vi "onCreated.vi"(8 "error in (no error)":errorcluster, 11 "Generator":refnum<class "Generator.lvclass">) -> (0 "error out":errorcluster, 3 "Generator out":refnum<class "Generator.lvclass">)   [LabVIEW 2019, in "Generator.lvclass"]
uses:
  Generator.lvclass
  <vilib>/JKI/JKI SMO/SMO/SMO.lvclass
panel:
  # "For instructions on how to use the JKI State Machine Objects, examples and video tutorials, visit:\nhttp://jki.net/state-machine-objects/\n\nJKI State Machine Objects™\nhttp://jki.net/state-machine-objects/\nCopyright (C) 2005-2015, JKI <info@jki.net>\nALL RIGHTS RESERVED"
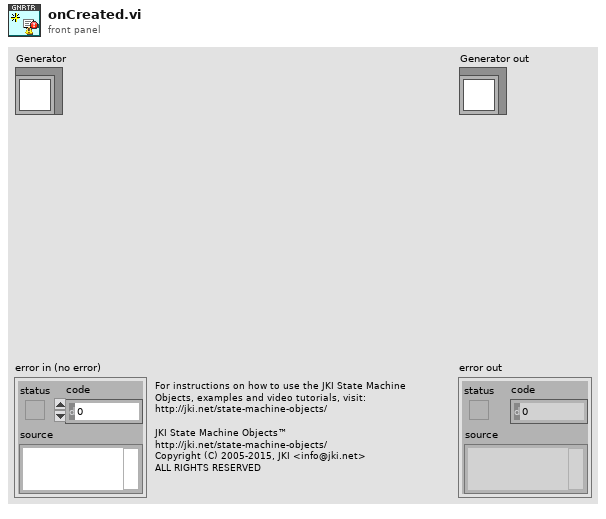
[diagram p1: front panel]
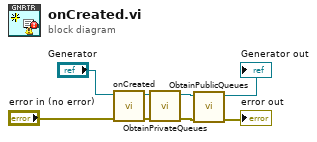
[diagram p0: block diagram]
diagram:
  n1 = call-parent "onCreated.vi"("error in (no error)"="error in (no error)", "SMO"="Generator") -> ("error out"=w5:errorcluster, "SMO out"=w6:refnum<class "Generator.lvclass">)  [unwired: 8 in]
  n2 = call "ObtainPrivateQueues.vi"("error in (no error)"=w5, "Generator"=w6) -> ("error out"=w3:errorcluster, "Generator out"=w4:refnum<class "Generator.lvclass">)  [unwired: 8 in]
  n3 = call "ObtainPublicQueues.vi"("error in (no error)"=w3, "Generator"=w4) -> ("error out"=→"error out":errorcluster, "Generator out"=→"Generator out":refnum<class "Generator.lvclass">)  [unwired: 8 in]
